vi "Write T Controller Settings.vi"(4 "New PID":cluster{"P":dbl, "I":dbl, "D":dbl}, 6 "Heater level":dbl, 7 "Set point":dbl, 8 "error in (no error)":errorcluster, 9 "New Heater mode":T1(ring), 10 "Heater range":dbl, 11 "Neocera LTC-21 in":refnum<class "Cryo-Con-22C.lvclass">) -> (0 "error out":errorcluster, 3 "Neocera LTC-21 out":refnum<class "Cryo-Con-22C.lvclass">)   [LabVIEW 2015, in "Cryo-Con-22C.lvclass"]
uses:
  Cryo-Con-22C.lvclass
  Instrument/Instrument.lvclass
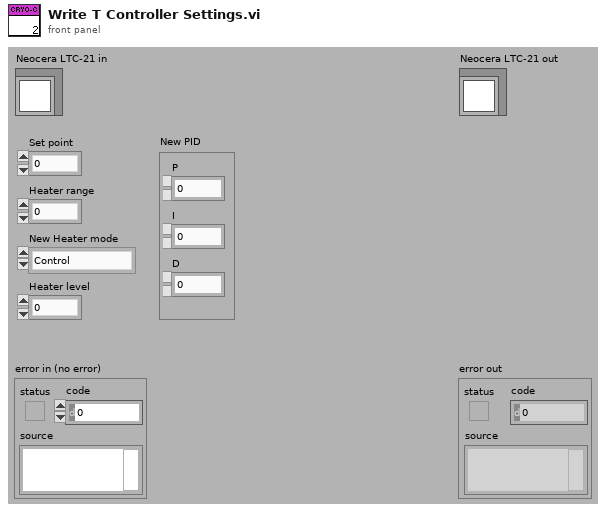
[diagram p1: front panel]
types:
  T1 = enum16{"Control", "Monitor", "Manual Heat", "Controller is in OFF mode", "Autotune is in progress"}
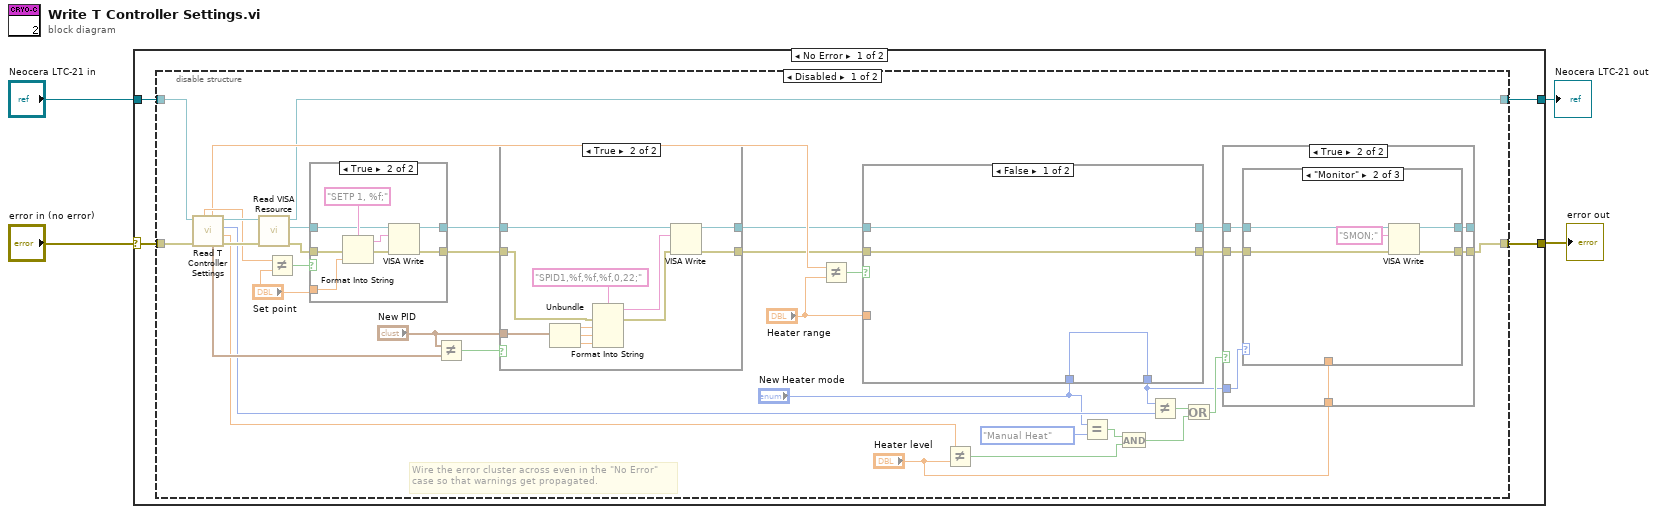
[diagram p0: block diagram]
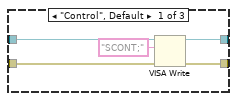
[diagram p4: hidden frame]
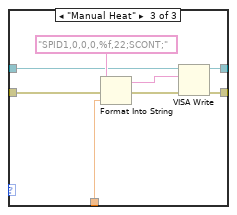
[diagram p5: hidden frame]
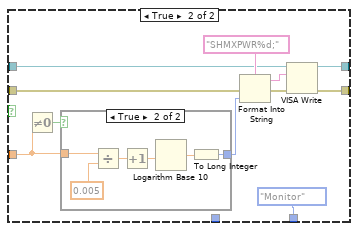
[diagram p6: hidden frame]
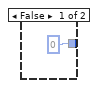
[diagram p7: hidden frame]
diagram:
  n1 = case shown="No Error" "error in (no error)" {
    selector: "error in (no error)" -> [w8 w116]
    tunnel: [w5 w116] -> w3
    tunnel: [w6 w115] -> w1
    tunnel: "Neocera LTC-21 in" -> [w7 w115]
    frame No Error {
      n2 = disable-structure shown="Disabled" {
        disable-tunnel: w8 -> [w32 w113]
        disable-tunnel: w7 -> [w31 w114]
        disable-tunnel: [w30 w114] -> w6
        disable-tunnel: [w26 w113] -> w5
        frame Disabled {
          # "Wire the error cluster across even in the \"No Error\"\ncase so that warnings get propagated."
          n3 = call-dynamic "Read T Controller Settings.vi"("error in (no error)"=w32, "Neocera LTC-21 in"=w31) -> ("error out"=w41:errorcluster, "Heater level"=w18:dbl, "Heater mode"=w15:T1, "Neocera LTC-21 out"=w42:refnum<class "Cryo-Con-22C.lvclass">, "PID"=w25:cluster{"P":dbl, "I":dbl, "D":dbl}, "Hater range"=w34:dbl, "Set point"=w40:dbl)  [unwired: 3 in]
          n4 = call "Read VISA Resource.vi"("error in (no error)"=w41, "Instrument.lvclass in"=w42) -> ("error out"=w38:errorcluster, "VISA Resource"=w36:refnum<visa-resource-name>, "Instrument.lvclass out"=w30:refnum<class "Cryo-Con-22C.lvclass">)  [unwired: 7 out]
          n5 = Not Equal?(x=w40, y="Set point") -> (x != y?=w39:bool)
          n6 = case shown="True" w39 {
            tunnel: w38 -> [w104 w110]
            tunnel: "Set point" -> [_ w111]
            tunnel: w36 -> [w103 w108]
            tunnel: [w104 w107] -> w23
            tunnel: [w103 w106] -> w21
            frame False {
            }
            frame True {
              n7 = Format Into String(format string="SETP 1, %f;" ("write buffer"), error in=w110, w111) -> (resulting string=w105:string, error out=w109:errorcluster)  [unwired: 1 in]
              n8 = VISA Write(VISA resource name=w108, write buffer=w105, error in (no error)=w109) -> (VISA resource name out=w106:refnum<visa-resource-name>, error out=w107:errorcluster)  [unwired: 1 out]
            }
          }
          n9 = Not Equal?(x="New PID", y=w25) -> (x != y?=w24:bool)
          n10 = case shown="True" w24 {
            tunnel: w23 -> [w44 w50]
            tunnel: [w44 w48] -> w22
            tunnel: w21 -> [w43 w45]
            tunnel: [w43 w47] -> w20
            tunnel: "New PID" -> [_ w55]
            frame False {
            }
            frame True {
              n11 = Unbundle(w55) -> ("P"=w54:dbl, "I"=w53:dbl, "D"=w52:dbl)
              n12 = Format Into String(format string="SPID1,%f,%f,%f,0,22;", error in=w50, w54, w53, w52) -> (resulting string=w46:string, error out=w49:errorcluster)  [unwired: 1 in]
              n13 = VISA Write(VISA resource name=w45, write buffer=w46, error in (no error)=w49) -> (VISA resource name out=w47:refnum<visa-resource-name>, error out=w48:errorcluster)  [unwired: 1 out]
            }
          }
          n14 = Not Equal?(x=w34, y="Heater range") -> (x != y?=w35:bool)
          n15 = case shown="False" w35 {
            tunnel: w22 -> [w84 w94]
            tunnel: "Heater range" -> [_ w88]
            tunnel: w20 -> [w83 w92]
            tunnel: [w84 w91] -> w27
            tunnel: [w83 w90] -> w28
            tunnel: [w82 T1."Monitor" ("New Heater mode")] -> w10
            tunnel: "New Heater mode" -> [w82 _]
            frame False {
            }
            frame True {
              n16 = Not Equal To 0?(x=w88) -> (x != 0?=w89:bool)
              n17 = case shown="True" w89 {
                tunnel: w88 -> [_ w101]
                tunnel: [0 w98] -> w87
                frame False {
                }
                frame True {
                  n18 = Divide(x=w101, y=0.005) -> (x/y=w100:dbl)
                  n19 = Increment(x=w100) -> (x+1=w97:dbl)
                  n20 = Logarithm Base 10(1:w97) -> (0:w99:dbl)
                  n21 = To Long Integer(number=w99) -> (32bit integer=w98:i32)
                }
              }
              n22 = Format Into String(format string="SHMXPWR%d;" ("write buffer"), error in=w94, w87) -> (resulting string=w86:string, error out=w93:errorcluster)  [unwired: 1 in]
              n23 = VISA Write(VISA resource name=w92, write buffer=w86, error in (no error)=w93) -> (VISA resource name out=w90:refnum<visa-resource-name>, error out=w91:errorcluster)  [unwired: 1 out]
            }
          }
          n24 = Not Equal?(x=w18, y="Heater level") -> (x != y?=w13:bool)
          n25 = Equal?(x="New Heater mode", y=T1."Manual Heat" ("New Heater mode")) -> (x = y?=w14:bool)
          n26 = And(x=w14, y=w13) -> (x .and. y?=w11:bool)
          n27 = Not Equal?(x=w10, y=w15) -> (x != y?=w33:bool)
          n28 = Or(x=w33, y=w11) -> (x .or. y?=w12:bool)
          n29 = case shown="True" w12 {
            tunnel: w10 -> [_ w63]
            tunnel: w27 -> [w57 w62]
            tunnel: w28 -> [w56 w61]
            tunnel: [w56 w60] -> _
            tunnel: [w57 w59] -> w26
            tunnel: "Heater level" -> [_ w58]
            frame False {
            }
            frame True {
              n30 = case shown="\"Monitor\"" w63 {
                tunnel: w62 -> [w68 w73 w79]
                tunnel: w61 -> [w67 w72 w75]
                tunnel: [w65 w70 w78] -> w59
                tunnel: [w64 w69 w74] -> w60
                tunnel: w58 -> [_ _ w76]
                frame "Control", Default {
                  n31 = VISA Write(VISA resource name=w67, write buffer="SCONT;", error in (no error)=w68) -> (VISA resource name out=w64:refnum<visa-resource-name>, error out=w65:errorcluster)  [unwired: 1 out]
                }
                frame "Monitor" {
                  n32 = VISA Write(VISA resource name=w72, write buffer="SMON;", error in (no error)=w73) -> (VISA resource name out=w69:refnum<visa-resource-name>, error out=w70:errorcluster)  [unwired: 1 out]
                }
                frame "Manual Heat" {
                  n33 = Format Into String(format string="SPID1,0,0,0,%f,22;SCONT;", error in=w79, w76) -> (resulting string=w80:string, error out=w81:errorcluster)  [unwired: 1 in]
                  n34 = VISA Write(VISA resource name=w75, write buffer=w80, error in (no error)=w81) -> (VISA resource name out=w74:refnum<visa-resource-name>, error out=w78:errorcluster)  [unwired: 1 out]
                }
              }
            }
          }
        }
        frame Enabled {
        }
      }
    }
    frame Error {
    }
  }
  "error out" <- w3
  "Neocera LTC-21 out" <- w1
